vi "Search Device.vi"() -> ()   [LabVIEW 2015]
uses:
  RTL-SDR Class/RTL-SDR.lvclass
  RTL-SDR Class/TypeDef/Device USB String.ctl
panel:
  out "error out":errorcluster
  out "function return":i32
  out "Device USB Strings":T1
  in  "stop":bool
  in  "Device Index":u32
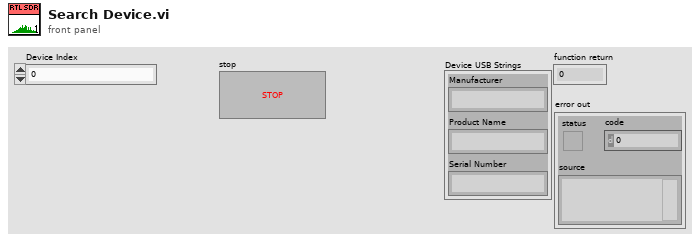
[diagram p1: front panel]
types:
  T1 = typedef "RTL-SDR.lvclass/Device USB String.ctl" = cluster{"Manufacturer":string, "Product Name":string, "Serial Number":string}
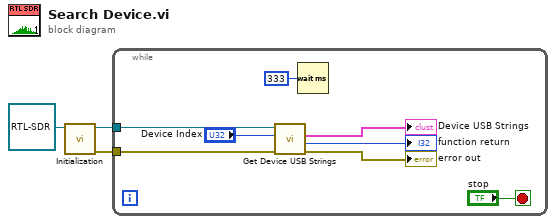
[diagram p0: block diagram]
diagram:
  n1 = call "Initialization.vi"("RTL-SDR in"=refnum<class "RTL-SDR.lvclass"> refnum) -> ("error out"=w2:errorcluster, "RTL-SDR out"=w3:refnum<class "RTL-SDR.lvclass">)  [unwired: 8 in, 1 out]
  n2 = while {
    tunnel: w3 -> [w11]
    tunnel: w2 -> [w10]
    stop <- "stop" stop-if-true
    n3 = call "Get Device USB Strings.vi"("error in (no error)"=w10, "Device Index"="Device Index", "RTL-SDR in"=w11) -> ("error out"=→"error out":errorcluster, "function return"=→"function return":i32, "Device USB Strings"=→"Device USB Strings":T1)  [unwired: 5 in, 1 out]
    n4 = Wait (ms)(milliseconds to wait=u32 333) -> ()  [unwired: 1 out]
  }
